vi "MultiRun Description.vi"() -> ()   [LabVIEW 2016]
uses:
  ADAM Client/Sub VIs/ADAM Controls/Module_type_ADAM.ctl
  ADAM Client/Sub VIs/ADAM Controls/Update_scan_value.ctl
  ADAM Client/Sub VIs/ADAM Controls/Calib_type_ADAM.ctl
  Globals/Preference_global.vi
panel:
  in  "OK":bool
  out "Channel Name":string
  in  "Previous Messages":u16(ring) items=["Run 2", "Run 1"]
  in  "Please add a Multi Run Description.":string
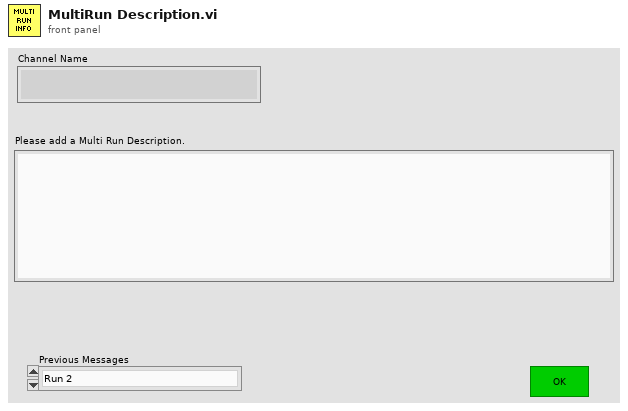
[diagram p1: front panel]
types:
  T1 = typedef "Update_scan_value.ctl" = cluster{"Channel Name":string, "New Value":dbl}
  T2 = typedef "Module_type_ADAM.ctl" = string
  T3 = typedef "Ch_description_ADAM.ctl" = cluster{"Ch Name":string, "Type":T2, "Function":T4, "Ch State":T5, "Calibration type":T6, "A":dbl, "B":dbl, "C":dbl, "D":dbl, "Comments":string, "Address":T7, "String":string, "Duty":u16}
  T4 = typedef "Function_ADAM.ctl" = enum16{"Analogue Input", "Digital Input", "Event counter", "Event rate", "Analogue Output", "Digital Output", "Relay Output"}
  T5 = typedef "Channel_State.ctl" = enum16{"On", "Off", "Always On", "Always Off"}
  T6 = typedef "Calib_type_ADAM.ctl" = string
  T7 = typedef "Address.ctl" = cluster{"Main":i32, "Ch.":i32, "Sub":i32, "Port Name":string}
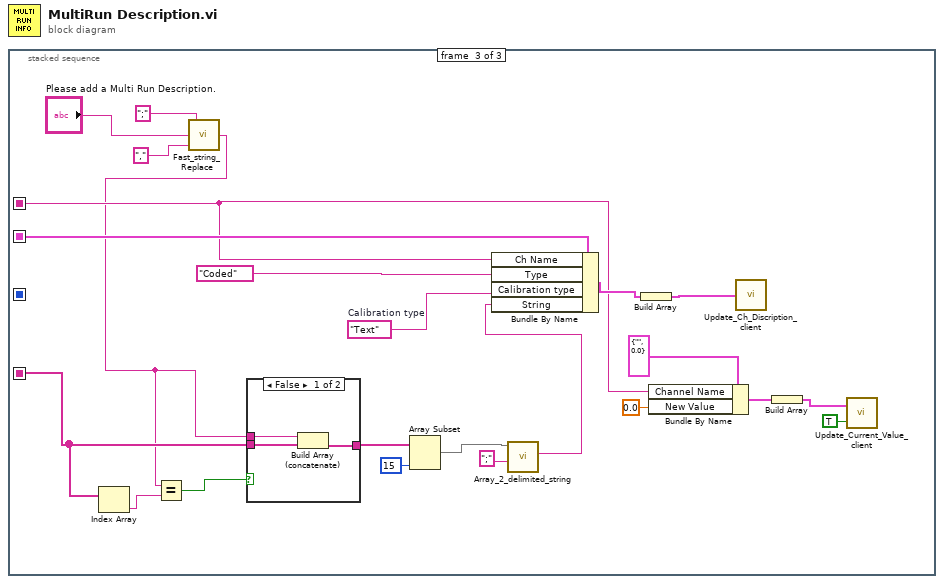
[diagram p0: block diagram]
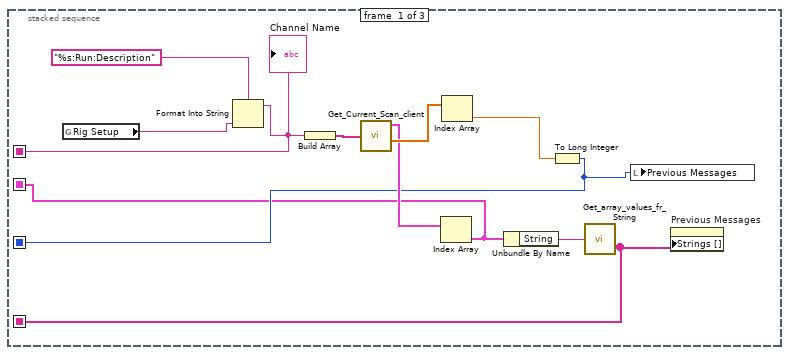
[diagram p2: hidden frame]
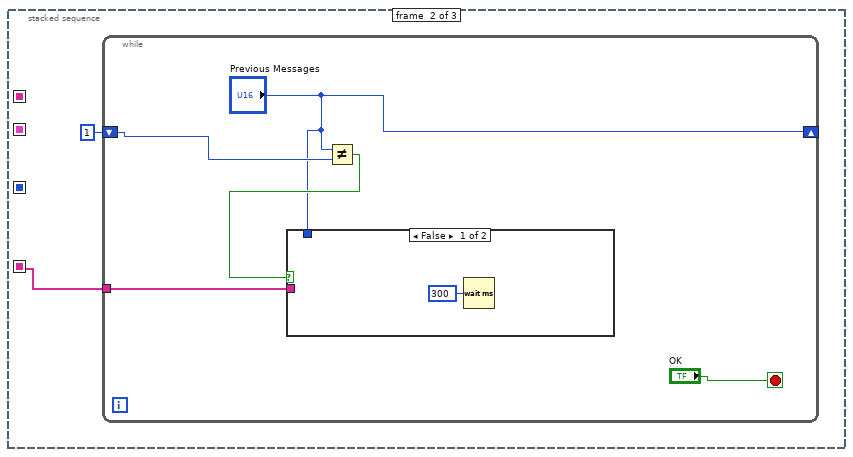
[diagram p3: hidden frame]
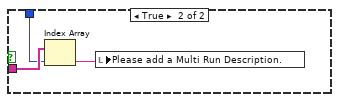
[diagram p4: hidden frame]
diagram:
  n1 = stacked-sequence {
    seq-local: [w5 _ _] -> [_ w13 w33]
    seq-local: [w3 _ _] -> [_ _ _]
    seq-local: [w2 _ _] -> [_ _ w45]
    seq-local: [w1 _ _] -> [_ _ w37]
    frame #0 {
      n2 = global read "Preference_global.vi" "Rig Setup"() -> (w11:string)
      n3 = Format Into String(format string="%s:Run:Description", w11) -> (resulting string=w1:string)  [unwired: 2 in, 1 out]
      "Channel Name" <- w1
      n4 = Build Array(w1) -> (w9:string[])
      n5 = call "Get_Current_Scan_client.vi"("ADAM Ch Names"=w9) -> ("Ch Description Array"=w7:T3[], "Numerical Values"=w8:dbl[])  [unwired: 1 in, 1 out]
      n6 = Index Array(array=w7) -> (element=w2:T3)  [unwired: 1 in]
      n7 = Index Array(array=w8) -> (element=w4:dbl)  [unwired: 1 in]
      n8 = Unbundle By Name(w2) -> ("String"=w6:string)
      n9 = To Long Integer(number=w4) -> (32bit integer=w3:i32)
      n10 = call "Get_array_values_fr_String.vi"("String Value"=w6) -> ("String array"=w5:string[])  [unwired: 1 out]
      n11 = local write "Previous Messages"(w3) -> ()
      n12 = property on="Previous Messages" class="Ring (strict)"("Strings []"=w5) -> ()  [unwired: 2 in, 2 out]
    }
    frame #1 {
      n13 = while {
        shift-right: ["Previous Messages"] -> _
        shift-left: u16 1 ("Previous Messages") -> [w18]
        tunnel: w13 -> [w16]
        stop <- "OK" stop-if-true
        n14 = Not Equal?(x="Previous Messages", y=w18) -> (x != y?=w17:bool)
        n15 = case shown="False" w17 {
          tunnel: w16 -> [_ w21]
          tunnel: "Previous Messages" -> [_ w20]
          frame False {
            n16 = Wait (ms)(milliseconds to wait=u32 300) -> ()  [unwired: 1 out]
          }
          frame True {
            n17 = Index Array(array=w21, index=w20) -> (element=w22:string)
            n18 = local write "Please add a Multi Run Description."(w22) -> ()
          }
        }
      }
    }
    frame #2 {
      w23 = T6 "Text"  # Calibration type
      n19 = Index Array(array=w33) -> (element=w32:string)  [unwired: 1 in]
      n20 = call "Fast_string_Replace.vi"("Replace match with:"=",", "Input String"="Please add a Multi Run Description.", "regular expression"=";") -> ("Output String"=w24:string)  [unwired: 1 in, 1 out]
      n21 = Equal?(x=w24, y=w32) -> (x = y?=w31:bool)
      n22 = case shown="False" w31 {
        tunnel: [w48 w49] -> w30
        tunnel: w33 -> [w47 w49]
        tunnel: w24 -> [w46 _]
        frame False {
          n23 = Build Array (concatenate)(w46, w47) -> (w48:string[])
        }
        frame True {
        }
      }
      n24 = Array Subset(array=w30, length=15) -> (w29:string[])  [unwired: 1 in]
      n25 = call "Array_2_delimited_string.vi"("delimiter (Tab)"=";", "Array of Strings"=w29) -> ("delimited string"=w42:string)  [unwired: 9 in]
      n26 = Bundle By Name(cluster=w45, "Ch Name"=w37, "Type"=T2 "Coded", "Calibration type"=w23, "String"=w42) -> (w41:T3)
      n27 = Build Array(w41) -> (w40:T3[])
      n28 = Bundle By Name(cluster=T1 {"Channel Name"="", "New Value"=0.0} ("Update Scan Value Cluster"), "Channel Name"=w37, "New Value"=0.0) -> (w35:T1)
      n29 = call "Update_Ch_Discription_client.vi"("Channels to update In"=w40) -> ()  [unwired: 1 in]
      n30 = Build Array(w35) -> (w34:T1[])
      n31 = call "Update_Current_Value_client.vi"("Don't Bother with check?"=TRUE, "Update array in"=w34) -> ()
    }
  }
